vi "Analog Replays Page - Multi FPGA.vi"(8 "error in (no error)":errorcluster, 11 "Node Ptr":T1 format="%.0x") -> (0 "error out":errorcluster)   [LabVIEW 2015, in "Engine Simulation Toolkit System Explorer.lvlib"]
uses:
  Engine Simulation Toolkit System Explorer.lvlib
  <vilib>/NI Veristand/Custom Device API/Custom Device Item Ref.ctl
  Shared/Properties.vi
  Shared/Constants and GUIDs.vi
  <vilib>/NI Veristand/Custom Device API/Get Item Property (String Array).vi
  <vilib>/NI Veristand/Custom Device API/Custom Device API.lvlib
  Shared/Engine Simulation Toolkit Shared.lvlib
  <vilib>/NI Veristand/Custom Device Tools/Custom Device Utility Library/Custom Device Utility Library.lvlib
panel:
  in  "remove":bool
  in  "add":bool
  in  "Replay listbox":i32[](listbox) caption="Available Analog Replays"
  in  "Header":cluster{"Section Name":string}={"Section Name"="Analog Replays Settings"}
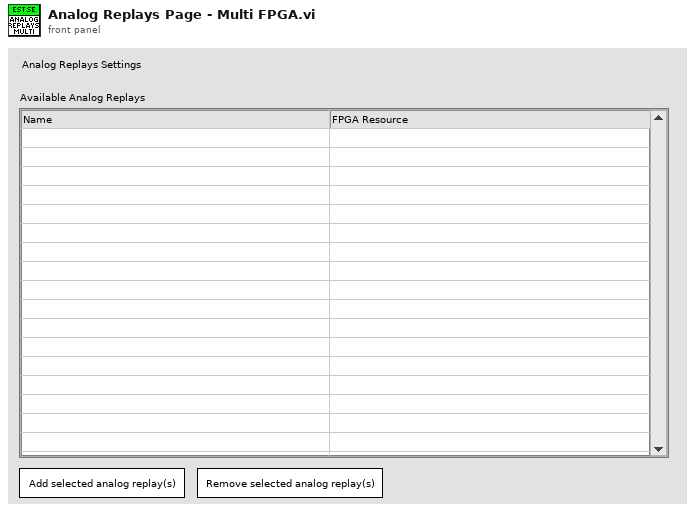
[diagram p1: front panel]
types:
  T1 = typedef "Custom Device API.lvlib/Custom Device Item Ref.ctl" = u64
  T2 = enum8{"Enabled", "Disabled", "Disabled and Grayed Out"}
  T3 = cluster{"ip list property name":string, string[]}[]
  T4 = typedef "Custom Device API.lvlib/Custom Device Commands.ctl" = enum16{"Default", "Item renamed", "Shutdown", "Dynamic button pressed"}
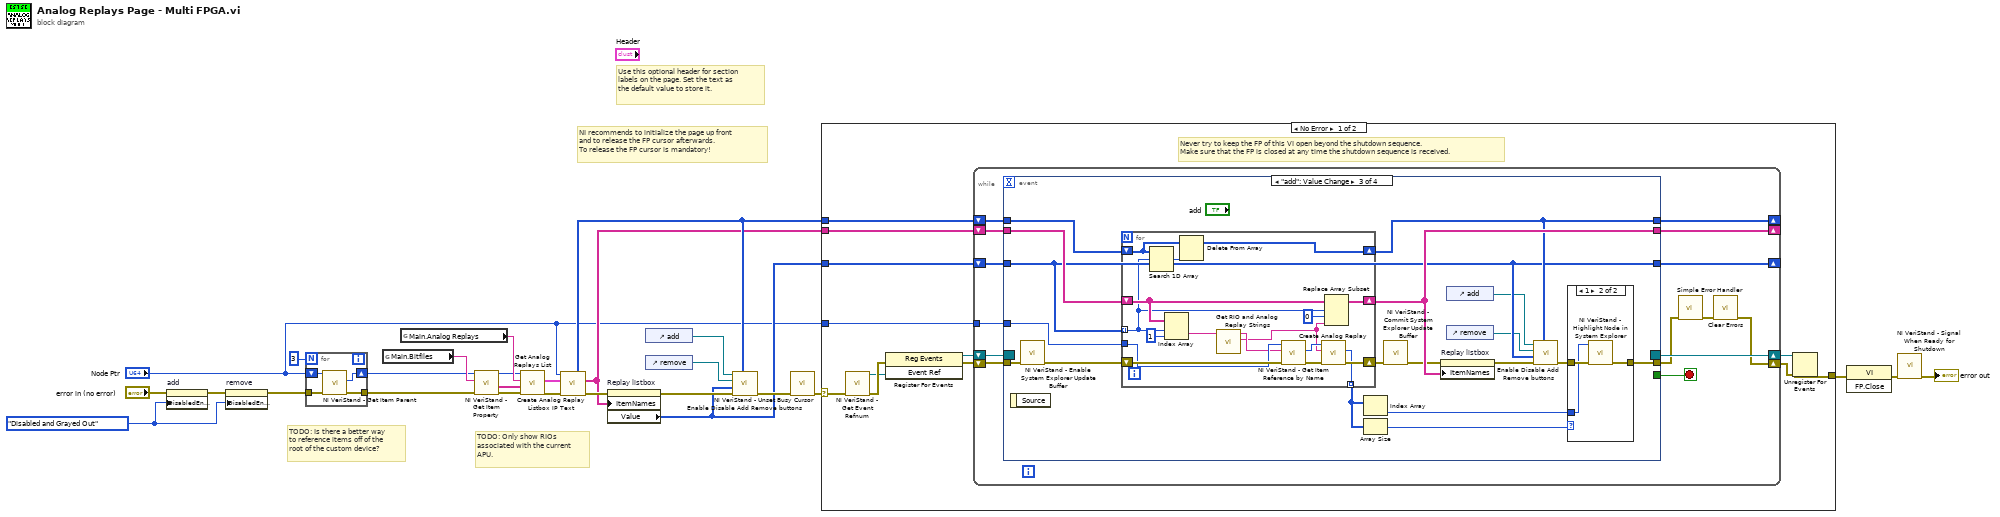
[diagram p0: block diagram]
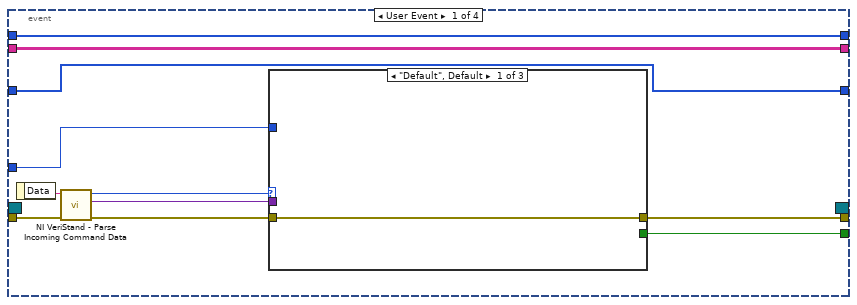
[diagram p2: hidden frame]
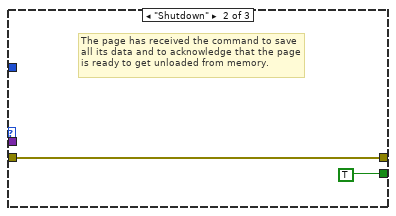
[diagram p3: hidden frame]
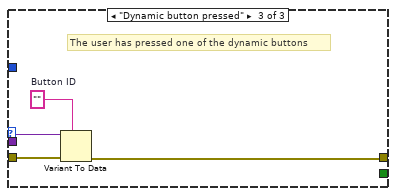
[diagram p4: hidden frame]
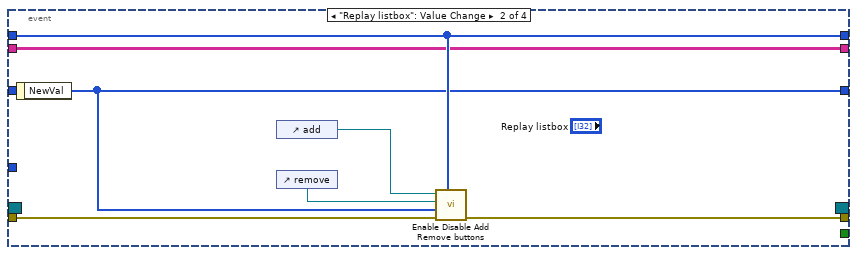
[diagram p5: hidden frame]
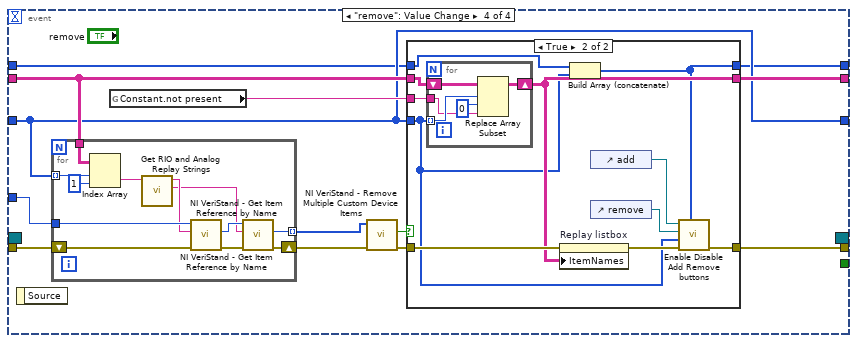
[diagram p7: hidden frame]
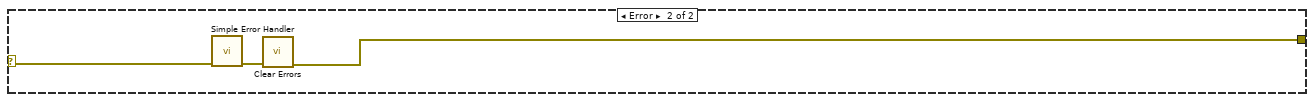
[diagram p9: hidden frame]
diagram:
  w18 = T2."Disabled and Grayed Out" ("Disabled")
  # "TODO: Only show RIOs\nassociated with the current\nAPU."
  # "TODO: Is there a better way\nto reference items off of the\nroot of the custom device?"
  # "Use this optional header for section labels on the page. Set the text as the default value to store it."
  # "NI recommends to initialize the page up front\nand to release the FP cursor afterwards.\nTo release the FP cursor is mandatory!"
  n1 = property on="add" class="Bool"(error in="error in (no error)", "DisabledEnum"=w18) -> (error out=w19:errorcluster)  [unwired: 1 in, 1 out]
  n2 = property on="remove" class="Bool"(error in=w19, "DisabledEnum"=w18) -> (error out=w3:errorcluster)  [unwired: 1 in, 1 out]
  n3 = for {
    N: 3 -> [_]
    tunnel: [w31] -> w5
    tunnel: w3 -> [w30]
    shift-right: [w28] -> w2
    shift-left: "Node Ptr" -> [w29]
    n4 = call <vilib>:"NI VeriStand - Get Item Parent.vi"("error in (no error)"=w30, "Item Ref in"=w29) -> ("error out"=w31:errorcluster, "Parent Ref"=w28:T1)  [unwired: 6 in, 2 out]
  }
  n5 = global read "Properties.vi" "Main.Bitfiles"() -> (w9:string)
  n6 = global read "Properties.vi" "Main.Analog Replays"() -> (w21:string)
  n7 = call-poly <vilib>:"NI VeriStand - Get Item Property.vi"("error in (no error)"=w5, "Property Name"=w9, "Item Ref in"=w2) -> ("error out"=w11:errorcluster, "Value"=w6:string[], "Item Ref out"=w10:T1)  [unwired: 5 in, 1 out]
  n8 = call "Get Analog Replays List.vi"("error in (no error)"=w11, "rio names"=w6, "ip list property name"=w21, "Item Ref in"=w10) -> ("error out"=w23:errorcluster, "rios and analog replays"=w8:T3)  [unwired: 5 in, 1 out]
  n9 = call "Create Analog Replay Listbox IP Text.vi"("error in (no error)"=w23, "rios and analog replays"=w8, "Section Ref in"="Node Ptr") -> ("error out"=w20:errorcluster, "listbox text"=w7:string[][], "not present item indexes"=w13:i32[])  [unwired: 5 in, 1 out]
  n10 = property on="Replay listbox" class="MCListbox (strict)"(error in=w20, "ItemNames"=w7) -> (error out=w15:errorcluster, "Value"=w12:i32[])  [unwired: 1 in, 1 out]
  n11 = control-ref of="add"() -> (w16:refnum<vi>)
  n12 = control-ref of="remove"() -> (w17:refnum<vi>)
  n13 = call "Enable Disable Add Remove buttons.vi"("not present item indexes"=w13, "error in (no error)"=w15, "selected items"=w12, "remove button"=w17, "add button"=w16) -> ("error out"=w14:errorcluster)  [unwired: 6 in]
  n14 = call <vilib>:"NI VeriStand - Unset Busy Cursor.vi"("error in (no error)"=w14) -> ("error out"=w24:errorcluster)  [unwired: 10 out]
  n15 = case shown="No Error" w24 {
    selector: w24 -> [w35 w168]
    tunnel: [w40 w166] -> w27
    tunnel: "Node Ptr" -> [w36 _]
    tunnel: w7 -> [w34 _]
    tunnel: w13 -> [w33 _]
    tunnel: w12 -> [w32 _]
    frame No Error {
      # "Never try to keep the FP of this VI open beyond the shutdown sequence.\nMake sure that the FP is closed at any time the shutdown sequence is received."
      n16 = call <vilib>:"NI VeriStand - Get Event Refnum.vi"("error in (no error)"=w35) -> ("error out"=w43:errorcluster, "Event Ref"=w39:refnum<user-event>)  [unwired: 9 out]
      n17 = register-events(error in=w43, w39) -> (reference out=w37:refnum<event-registration>, error out=w38:errorcluster)  [unwired: 1 in]
      n18 = while {
        tunnel: w36 -> [w53]
        shift-right: [w50] -> w41
        shift-left: w38 -> [w56]
        shift-right: [w57] -> w42
        shift-left: w37 -> [w55]
        shift-right: [w48] -> _
        shift-left: w32 -> [w45]
        shift-right: [w46] -> _
        shift-left: w33 -> [w44]
        shift-right: [w47] -> _
        shift-left: w34 -> [w49]
        stop <- w54 stop-if-true
        n19 = event shown="[2] \"add\": Value Change" {
          selector: w55 -> [_ _ _ _]
          dyn-events: [_ _ _ _] -> w57
          timeout: _ -> [_ _ _ _]
          tunnel: w56 -> [w68 w82 w100 w133]
          tunnel: [w64 _ _ _] -> w54
          tunnel: [w63 w81 w85 w134] -> w52
          tunnel: w53 -> [w62 _ w99 w132]
          tunnel: w49 -> [w59 w76 w98 w127]
          tunnel: w44 -> [w58 w78 w97 w123]
          tunnel: [w60 w77 w92 w124] -> w48
          tunnel: w45 -> [w60 _ w92 w124]
          tunnel: [w59 w76 w95 w125] -> w47
          tunnel: [w58 w78 w93 w122] -> w46
          event User Event {
            n20 = event-data() -> ("Data"=w67:string)  [unwired: 1 out]
            n21 = call <vilib>:"NI VeriStand - Parse Incoming Command Data.vi"("error in (no error)"=w68, "Incoming data"=w67) -> ("error out"=w66:errorcluster, "Outgoing data"=w61:variant, "Action"=w65:T4)  [unwired: 7 out]
            n22 = case shown="\"Default\", Default" w65 {
              tunnel: w66 -> [w69 w70 w75]
              tunnel: [_ TRUE _] -> w64
              tunnel: [w69 w70 w72] -> w63
              tunnel: w62 -> [_ _ _]
              tunnel: w61 -> [_ _ w74]
              frame "Default", Default {
              }
              frame "Shutdown" {
                # "The page has received the command to save all its data and to acknowledge that the page is ready to get unloaded from memory."
              }
              frame "Dynamic button pressed" {
                w73 = ""  # Button ID
                # "The user has pressed one of the dynamic buttons"
                n23 = Variant To Data(error in=w75, type=w73, Variant=w74) -> (error out=w72:errorcluster)  [unwired: 1 out]
              }
            }
          }
          event "Replay listbox": Value Change {
            n24 = event-data() -> ("NewVal"=w77:i32[])  [unwired: 1 out]
            n25 = control-ref of="add"() -> (w80:refnum<vi>)
            n26 = control-ref of="remove"() -> (w79:refnum<vi>)
            n27 = call "Enable Disable Add Remove buttons.vi"("not present item indexes"=w78, "error in (no error)"=w82, "selected items"=w77, "remove button"=w79, "add button"=w80) -> ("error out"=w81:errorcluster)  [unwired: 6 in]
          }
          event "add": Value Change {
            n28 = event-data() -> ()  [unwired: 2 out]
            n29 = call <vilib>:"NI VeriStand - Enable System Explorer Update Buffer.vi"("error in (no error)"=w100) -> ("error out"=w88:errorcluster)  [unwired: 10 in]
            n30 = for {
              tunnel: w99 -> [w109]
              shift-right: [w121] -> w96
              shift-left: w88 -> [w111]
              tunnel: w92 -> [w116] mode=indexing
              shift-right: [w118] -> w95
              shift-left: w98 -> [w119]
              shift-right: [w113] -> w93
              shift-left: w97 -> [w115]
              tunnel: [w112] -> w87 mode=indexing
              n31 = Search 1D Array(1D array=w115, element=w116) -> (index of element=w114:i32)  [unwired: 1 in]
              n32 = Index Array(array=w119, index (row)=w116, index (col)=1 ("disabled index (col)")) -> (element=w105:string)
              n33 = Delete From Array(array=w115, index=w114) -> (array with subset deleted=w113:i32[])  [unwired: 1 in, 1 out]
              n34 = call "Get RIO and Analog Replay Strings.vi"("rio/analog replay"=w105) -> ("analog replay"=w106:string, "rio"=w107:string)  [unwired: 9 in]
              n35 = call <vilib>:"NI VeriStand - Get Item Reference by Name.vi"("error in (no error)"=w111, "Item Name"=w107, "Parent Ref in"=w109) -> ("error out"=w110:errorcluster, "Item Ref"=w108:T1)  [unwired: 5 in, 2 out]
              n36 = call "Create Analog Replay.vi"("error in (no error)"=w110, "analog replay name"=w106, "Section Ptr"=w108) -> ("error out"=w121:errorcluster, "Analog replay ref"=w112:T1)  [unwired: 6 in, 1 out]
              n37 = Replace Array Subset(array=w119, new element=w106, index (row)=w116, index (col)=0 ("disabled index (col)")) -> (w118:string[][])
            }
            n38 = Index Array(array=w87) -> (element=w83:T1)  [unwired: 1 in]
            n39 = Array Size(array=w87) -> (size(s)=w86:i32)
            n40 = call <vilib>:"NI VeriStand - Commit System Explorer Update Buffer.vi"("error in (no error)"=w96) -> ("error out"=w89:errorcluster)  [unwired: 10 in]
            n41 = property on="Replay listbox" class="MCListbox (strict)"(error in=w89, "ItemNames"=w95) -> (error out=w94:errorcluster)  [unwired: 1 in, 1 out]
            n42 = control-ref of="add"() -> (w91:refnum<vi>)
            n43 = control-ref of="remove"() -> (w90:refnum<vi>)
            n44 = call "Enable Disable Add Remove buttons.vi"("not present item indexes"=w93, "error in (no error)"=w94, "selected items"=w92, "remove button"=w90, "add button"=w91) -> ("error out"=w84:errorcluster)  [unwired: 6 in]
            n45 = case shown="1" w86 {
              tunnel: [w101 w103] -> w85
              tunnel: w84 -> [w101 w104]
              tunnel: w83 -> [_ w102]
              frame Default {
              }
              frame 1 {
                n46 = call <vilib>:"NI VeriStand - Highlight Node in System Explorer.vi"("error in (no error)"=w104, "Item Ref in"=w102) -> ("error out"=w103:errorcluster)  [unwired: 8 in, 1 out]
              }
            }
          }
          event "remove": Value Change {
            n47 = event-data() -> ()  [unwired: 2 out]
            n48 = for {
              tunnel: w124 -> [w164] mode=indexing
              tunnel: w127 -> [w165]
              tunnel: w132 -> [w162]
              tunnel: [w156] -> w130 mode=indexing
              shift-right: [w157] -> w131
              shift-left: w133 -> [w163]
              n49 = Index Array(array=w165, index (row)=w164, index (col)=1 ("disabled index (col)")) -> (element=w160:string)
              n50 = call "Get RIO and Analog Replay Strings.vi"("rio/analog replay"=w160) -> ("analog replay"=w154:string, "rio"=w159:string)  [unwired: 9 in]
              n51 = call <vilib>:"NI VeriStand - Get Item Reference by Name.vi"("error in (no error)"=w163, "Item Name"=w159, "Parent Ref in"=w162) -> ("error out"=w158:errorcluster, "Item Ref"=w155:T1)  [unwired: 5 in, 2 out]
              n52 = call <vilib>:"NI VeriStand - Get Item Reference by Name.vi"("error in (no error)"=w158, "Item Name"=w154, "Parent Ref in"=w155) -> ("error out"=w157:errorcluster, "Item Ref"=w156:T1)  [unwired: 5 in, 2 out]
            }
            n53 = global read "Constants and GUIDs.vi" "Constant.not present"() -> (w126:string)
            n54 = call <vilib>:"NI VeriStand - Remove Multiple Custom Device Items.vi"("error in (no error)"=w131, "Item Refs in"=w130) -> ("error out"=w129:errorcluster, "Deleted?"=w128:bool)  [unwired: 8 in]
            n55 = case shown="True" w128 {
              tunnel: [w136 w147] -> w134
              tunnel: w129 -> [w136 w144]
              tunnel: w124 -> [_ w139]
              tunnel: w127 -> [w137 w143]
              tunnel: w126 -> [_ w142]
              tunnel: [w137 w141] -> w125
              tunnel: w123 -> [w135 w140]
              tunnel: [w135 w138] -> w122
              frame False {
              }
              frame True {
                n56 = for {
                  tunnel: w139 -> [w151] mode=indexing
                  shift-right: [w152] -> w141
                  shift-left: w143 -> [w153]
                  tunnel: w142 -> [w149]
                  n57 = Replace Array Subset(array=w153, new element=w149, index (row)=w151, index (col)=0 ("disabled index (col)")) -> (w152:string[][])
                }
                n58 = property on="Replay listbox" class="MCListbox (strict)"(error in=w144, "ItemNames"=w141) -> (error out=w148:errorcluster)  [unwired: 1 in, 1 out]
                n59 = Build Array (concatenate)(w140, w139) -> (w138:i32[])
                n60 = control-ref of="add"() -> (w146:refnum<vi>)
                n61 = control-ref of="remove"() -> (w145:refnum<vi>)
                n62 = call "Enable Disable Add Remove buttons.vi"("not present item indexes"=w138, "error in (no error)"=w148, "selected items"=w139, "remove button"=w145, "add button"=w146) -> ("error out"=w147:errorcluster)  [unwired: 6 in]
              }
            }
          }
        }
        n63 = call <vilib>:"Simple Error Handler.vi"("error in (no error)"=w52) -> ("error out"=w51:errorcluster)  [unwired: 1 in, 7 out]
        n64 = call <vilib>:"Clear Errors.vi"("error in (no error)"=w51) -> ("error out"=w50:errorcluster)  [unwired: 1 in, 5 out]
      }
      n65 = Unregister For Events(event registration refnum=w42, error in=w41) -> (error out=w40:errorcluster)
    }
    frame Error {
      n66 = call <vilib>:"Simple Error Handler.vi"("error in (no error)"=w168) -> ("error out"=w167:errorcluster)  [unwired: 1 in, 7 out]
      n67 = call <vilib>:"Clear Errors.vi"("error in (no error)"=w167) -> ("error out"=w166:errorcluster)  [unwired: 1 in, 5 out]
    }
  }
  n68 = invoke class="VI" method="FP.Close"(error in=w27) -> (error out=w26:errorcluster)  [unwired: 2 in, 2 out]
  n69 = call <vilib>:"NI VeriStand - Signal When Ready for Shutdown.vi"("error in (no error)"=w26) -> ("error out"=→"error out":errorcluster)  [unwired: 10 out]
